vi "Demo.vi"() -> ()   [LabVIEW 2018, in "hashlib.lvlib"]
doc: "Examples of the hashlib functions.\n\nCreated by: Ryan Pacini"
uses:
  hashlib.lvlib
panel:
  in  "Tab":T1(tab)
  out "CRC-8":u8 format="%02x"
  in  "Data 8":string="123456789"
  in  "Initial 8":u8 format="%02x"
  in  "Poly 8":u8=7 format="%02x"
  in  "Xor Out 8":u8 format="%02x"
  in  "Reflect Input? 8":bool
  in  "Reflect Output? 8":bool
  in  "Data 16":string="123456789"
  out "CRC-16":u16 format="%04x"
  in  "Initial 16":u16 format="%04x"
  in  "Poly 16":u16=32773 format="%04x"
  in  "Reflect Input? 16":bool
  in  "Xor Out 16":u16 format="%04x"
  in  "Reflect Output? 16":bool
  out "CRC-32":u32 format="%08x"
  in  "Data 32":string="123456789"
  in  "Initial 32":u32=4294967295 format="%08x"
  in  "Poly 32":u32=79764919 format="%08x"
  in  "Xor Out 32":u32=4294967295 format="%08x"
  in  "Reflect Input? 32":bool=TRUE
  in  "Reflect Output? 32":bool=TRUE
  in  "Data md5":string="The dog jumped over the log"
  out "MD5 (16-bytes)":string
  out "MD5 (Hex String)":string
  out "String out":string
  in  "Base64 Encoded in":string="VGhlIGRvZyBqdW1wZWQgb3ZlciB0aGUgbG9n"
  out "Base64 Encoded out":string
  in  "String in":string="The dog jumped over the log"
  out "SHA-256 Hexlify out":string
  in  "Data in":string="The dog jumped over the log"
  out "SHA-256 out":u32[](array[numeric]) format="%08x"
  in  "Key in":string="Puppy"
  out "HMAC-SHA-256 Hexlify out":string
  in  "Data2 in":string="The dog jumped over the log"
  out "HMAC-SHA-256 out":u32[](array[numeric]) format="%08x"
  out "PBKDF2-SHA-256 Hexlify out":string
  out "PBKDF2-SHA-256 out":u32[](array[numeric]) format="%08x"
  in  "password in":string="GoodPuppy"
  in  "salt in":string="My very secret salt key"
  in  "iterations in":i32=1024
  out "client_final_message":string
  in  "user":string="bob"
  in  "password":string="SuperSecretPassword"
  out "client_first_message":string
  in  "server_first_message":string="r=rOprNGfwEbeRWgbNEkqO%hvYDpWUa2RaTCAfuxFIlj)hNlF$k0,s=W22ZaJ0SNY7soEsUEjb6gQ==,i=4096"
  # "CRC-8"
  # "Calculate the 8-bit Cyclic Redundancy Check (CRC-8)"
  # "https://crccalc.com/"
  # "Checksum"
  # "CRC-16"
  # "Calculate the 16-bit Cyclic Redundancy Check (CRC-16)"
  # "https://crccalc.com/"
  # "Checksum"
  # "CRC-32"
  # "Calculate the 32-bit Cyclic Redundancy Check (CRC-32)"
  # "https://crccalc.com/"
  # "Checksum"
  # "MD5"
  # "MD5 Message-Digest Algorithm"
  # "Checksum"
  # "Base64 encode / decode"
  # "Base64 encodes or decodes a string using printable characters"
  # "Encode"
  # "Decode"
  # "SHA-256 hash"
  # "SHA-256 hashes the data into a 256 bit number"
  # "Hash"
  # "HMAC-SHA-256 hash"
  # "HMAC-SHA-256 hashes data with a key."
  # "Hash"
  # "PBKDF2-SHA-256 hash"
  # "PBKDF2-SHA-256 hashes a password using a salt (i.e. unique key)\nwith N iterations of entropy"
  # "Hash"
  # "SCRAM-SHA-256 (FIRST & FINAL CLIENT MESSAGE)"
  # "SCRAM-SHA-256 generates the FIRST & FINAL client messages used for web authentication.\n(See block diagram for more information)"
  # "1. FIRST\nclient\nmessage"
  # "3. FINAL\nclient\nmessage"
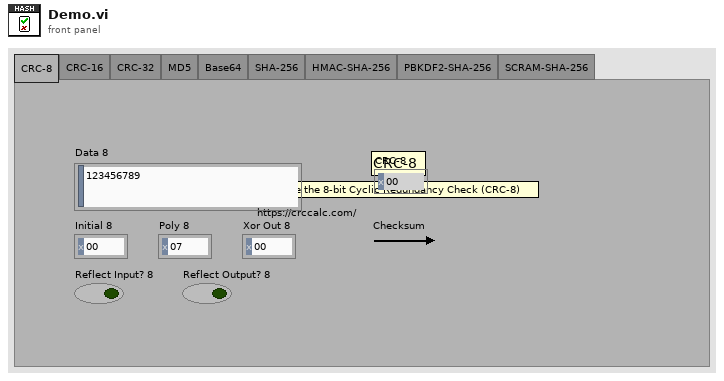
[diagram p1: front panel]
types:
  T1 = enum32{"CRC-8", "CRC-16", "CRC-32", "MD5", "Base64", "SHA-256", "HMAC-SHA-256", "PBKDF2-SHA-256", "SCRAM-SHA-256"}
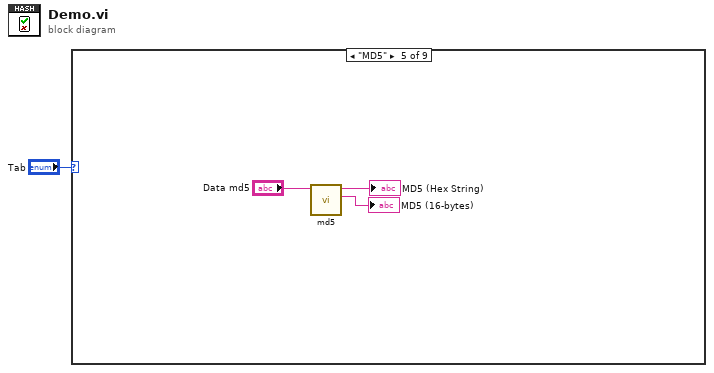
[diagram p0: block diagram]
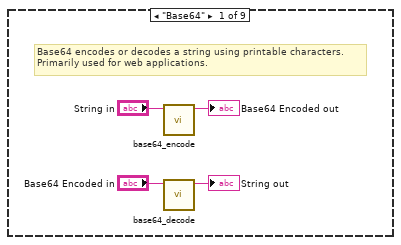
[diagram p2: hidden frame]
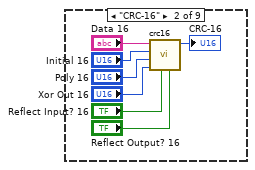
[diagram p3: hidden frame]
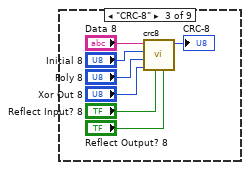
[diagram p4: hidden frame]
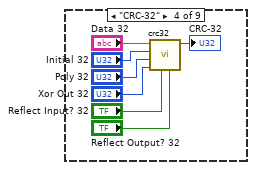
[diagram p5: hidden frame]
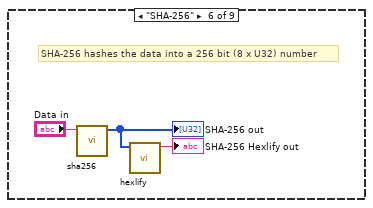
[diagram p6: hidden frame]
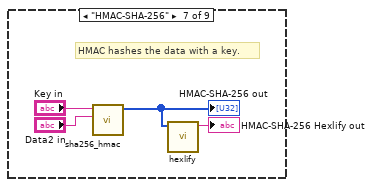
[diagram p7: hidden frame]
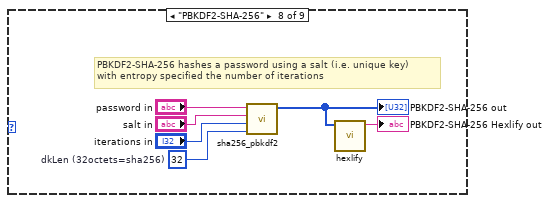
[diagram p8: hidden frame]
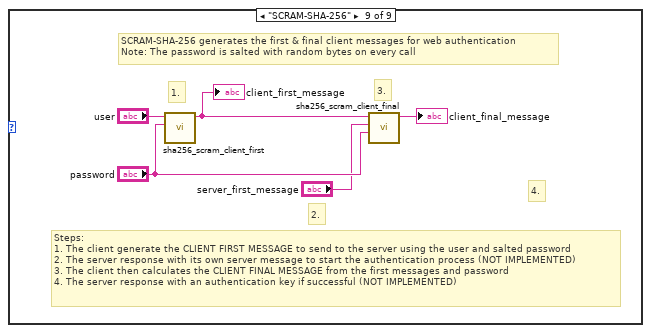
[diagram p9: hidden frame]
diagram:
  n1 = case shown="\"MD5\"" "Tab" {
    frame "Base64" {
      # "Base64 encodes or decodes a string using printable characters.\nPrimarily used for web applications."
      n2 = call "base64_encode.vi"("string"="String in") -> ("base64"=→"Base64 Encoded out":string)  [unwired: 10 in]
      n3 = call "base64_decode.vi"("base64"="Base64 Encoded in") -> ("string"=→"String out":string)  [unwired: 10 in]
    }
    frame "CRC-16" {
      n4 = call "crc16.vi"("Reflect Output? (F)"="Reflect Output? 16", "Reflect Input? (F)"="Reflect Input? 16", "Xor Out (0x0000)"="Xor Out 16", "Poly (0x8005)"="Poly 16", "Init (0x0000)"="Initial 16", "Data in"="Data 16") -> ("CRC-16"=→"CRC-16":u16)  [unwired: 5 in]
    }
    frame "CRC-8" {
      n5 = call "crc8.vi"("Reflect Output? (F)"="Reflect Output? 8", "Reflect Input? (F)"="Reflect Input? 8", "Xor Out (0x00)"="Xor Out 8", "Poly (0x07)"="Poly 8", "Init (0x00)"="Initial 8", "Data in"="Data 8") -> ("CRC-8"=→"CRC-8":u8)  [unwired: 5 in]
    }
    frame "CRC-32" {
      n6 = call "crc32.vi"("Reflect Output? (T)"="Reflect Output? 32", "Reflect Input? (T)"="Reflect Input? 32", "Xor Out (0xFFFFFFFF)"="Xor Out 32", "Poly (0x04C11DB7)"="Poly 32", "Init (0xFFFFFFFF)"="Initial 32", "Data in"="Data 32") -> ("CRC-32"=→"CRC-32":u32)  [unwired: 5 in]
    }
    frame "MD5" {
      n7 = call "md5.vi"("Data in"="Data md5") -> ("MD5 (16-bytes)"=→"MD5 (16-bytes)":string, "MD5 (Hex String)"=→"MD5 (Hex String)":string)  [unwired: 9 in]
    }
    frame "SHA-256" {
      # "SHA-256 hashes the data into a 256 bit (8 x U32) number"
      n8 = call "sha256.vi"("data"="Data in") -> ("sha256"=w31:u32[])  [unwired: 10 in]
      "SHA-256 out" <- w31
      n9 = call "hexlify.vi"("sha256"=w31) -> ("hex (0-9a-f)"=→"SHA-256 Hexlify out":string)  [unwired: 10 in]
    }
    frame "HMAC-SHA-256" {
      # "HMAC hashes the data with a key."
      n10 = call "sha256_hmac.vi"("data"="Data2 in", "key"="Key in") -> ("sha256"=w34:u32[])  [unwired: 9 in]
      "HMAC-SHA-256 out" <- w34
      n11 = call "hexlify.vi"("sha256"=w34) -> ("hex (0-9a-f)"=→"HMAC-SHA-256 Hexlify out":string)  [unwired: 10 in]
    }
    frame "PBKDF2-SHA-256" {
      w40 = 32  # dkLen (32octets=sha256)
      # "PBKDF2-SHA-256 hashes a password using a salt (i.e. unique key)\nwith entropy specified the number of iterations"
      n12 = call "sha256_pbkdf2.vi"("dkLen (32octets=sha256)"=w40, "iterations"="iterations in", "salt"="salt in", "password"="password in") -> ("sha-256"=w42:u32[])  [unwired: 7 in]
      "PBKDF2-SHA-256 out" <- w42
      n13 = call "hexlify.vi"("sha256"=w42) -> ("hex (0-9a-f)"=→"PBKDF2-SHA-256 Hexlify out":string)  [unwired: 10 in]
    }
    frame "SCRAM-SHA-256" {
      # "Steps:\n1. The client generate the CLIENT FIRST MESSAGE to send to the server using the user and salted password\n2. The server response with its own server message to start the authentication process (NOT IMPLEMENTED)\n3. The client then calculates the CLIENT FINAL MESSAGE from the first messages and password\n4. The server response with an authentication key if successful (NOT IMPLEMENTED)"
      # "4."
      # "3."
      # "2."
      # "1."
      # "SCRAM-SHA-256 generates the first & final client messages for web authentication\nNote: The password is salted with random bytes on every call"
      n14 = call "sha256_scram_client_first.vi"("password"="password", "user"="user") -> ("client_first_message"=w46:string)  [unwired: 9 in]
      "client_first_message" <- w46
      n15 = call "sha256_scram_client_final.vi"("password"="password", "server_first_message"="server_first_message", "client_first_message"=w46) -> ("client_final_message"=→"client_final_message":string)  [unwired: 8 in]
    }
  }
